vi "Check Reservation Groups Supported.vi"(8 "error in":errorcluster caption="error in (no error)") -> (0 "error out":errorcluster, 3 "use reservation groups?":bool)   [LabVIEW 2017, in "SLSC Switch Messaging.lvlib" / "SLSC Switch Consumer.lvclass"]
uses:
  SLSC Switch Consumer.lvclass
  <vilib>/nisyscfg/Get Installed Components.vi
  <vilib>/nisyscfg/Close (System).vi
  <vilib>/regexp/Match Regular Expression.xnode
  <vilib>/nisyscfg/nisyscfg.lvlib
  <vilib>/Utility/SystemLogging/NI_SystemLogging.lvlib
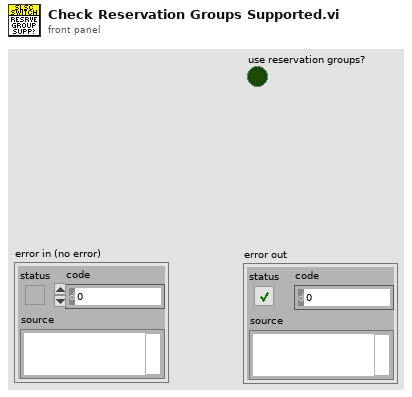
[diagram p1: front panel]
types:
  T1 = typedef "nisyscfg.lvlib/Software 1.2.ctl" = cluster{"title":string, "description":string, "ID":string, "version":string, "component type":T2}
  T2 = typedef "nisyscfg.lvlib/Component Type.ctl" = u32
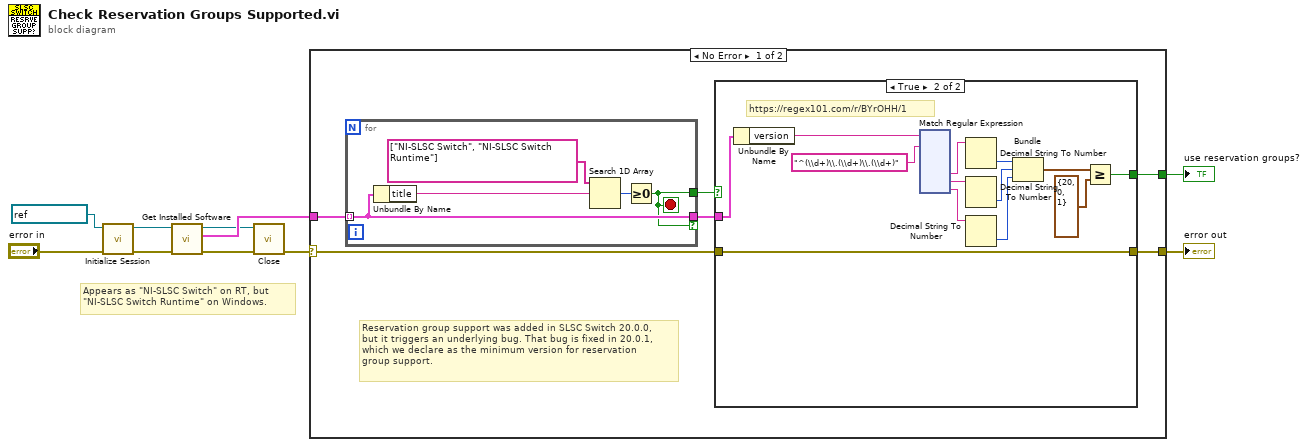
[diagram p0: block diagram]
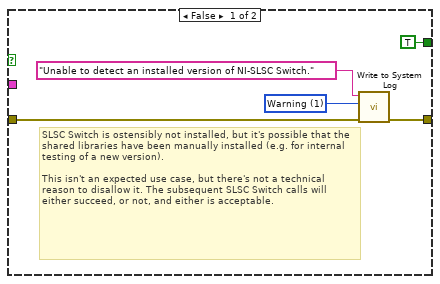
[diagram p2: hidden frame]
diagram:
  # "Appears as \"NI-SLSC Switch\" on RT, but\n\"NI-SLSC Switch Runtime\" on Windows."
  n1 = call <vilib>:"Initialize Session.vi"("error in (no error)"="error in", "Target (localhost)"=refnum<k21> "localhost") -> ("error out"=w9:errorcluster, "Session out"=w10:refnum<k21>)  [unwired: 8 in]
  n2 = call-poly <vilib>:"Get Installed Software.vi"("error in (no error)"=w9, "Session in"=w10) -> ("error out"=w6:errorcluster, "Software Components"=w8:T1[], "Session out"=w7:refnum<k21>)  [unwired: 7 in]
  n3 = call-poly <vilib>:"Close.vi"("error in (no error)"=w6, "Session in"=w7) -> ("error out"=w4:errorcluster)  [unwired: 9 in]
  n4 = case shown="No Error" w4 {
    selector: w4 -> [w12 w158]
    tunnel: w8 -> [w16 _]
    tunnel: [w13 _] -> w5
    tunnel: [w11 w158] -> w3
    frame No Error {
      # "Reservation group support was added in SLSC Switch 20.0.0,\nbut it triggers an underlying bug. That bug is fixed in 20.0.1,\nwhich we declare as the minimum version for reservation\ngroup support."
      n5 = for {
        tunnel: w16 -> [w157] mode=indexing
        tunnel: [w157] -> w14 if=w153
        tunnel: [w153] -> w15
        stop <- w153 stop-if-true
        n6 = Unbundle By Name(w157) -> ("title"=w155:string)
        n7 = Search 1D Array(1D array=string[] ["NI-SLSC Switch", "NI-SLSC Switch Runtime"], element=w155) -> (index of element=w154:i32)  [unwired: 1 in]
        n8 = Greater Or Equal To 0?(x=w154) -> (x >= 0?=w153:bool)
      }
      n9 = case shown="True" w15 {
        tunnel: [TRUE w26] -> w13
        tunnel: w14 -> [_ w27]
        tunnel: w12 -> [w19 w22]
        tunnel: [w18 w22] -> w11
        frame False {
          w20 = 1 items=["Error", "Warning", "Informational"] ("severity")
          # "SLSC Switch is ostensibly not installed, but it's possible that the shared libraries have been manually installed (e.g. for internal testing of a new version).\n\nThis isn't an expected use case, but there's not a technical reason to disallow it. The subsequent SLSC Switch calls will either succeed, or not, and either is acceptable."
          n10 = call <vilib>:"Write to System Log.vi"("error in (no error)"=w19, "severity"=w20, "message"="Unable to detect an installed version of NI-SLSC Switch.") -> ("error out"=w18:errorcluster)  [unwired: 8 in]
        }
        frame True {
          # "https://regex101.com/r/BYrOHH/1"
          n11 = Unbundle By Name(w27) -> ("version"=w23:string)
          n12 = xnode "Match Regular Expression"("input string"=w23, "regular expression"="^(\\d+)\\.(\\d+)\\.(\\d+)") -> ("submatch 1"=w29:string, "submatch 2"=w30:string, "submatch 3"=w31:string)  [unwired: 4 in, 5 out]
          n13 = Decimal String To Number(string=w29) -> (number=w32:i32)  [unwired: 2 in, 1 out]
          n14 = Decimal String To Number(string=w30) -> (number=w33:i32)  [unwired: 2 in, 1 out]
          n15 = Decimal String To Number(string=w31) -> (number=w34:i32)  [unwired: 2 in, 1 out]
          n16 = Bundle(w32, w33, w34) -> (w25:cluster{i32, i32, i32})  [unwired: 1 in]
          n17 = Greater Or Equal?(x=w25, y=cluster{i32, i32, i32} {20, 0, 1}) -> (x >= y?=w26:bool)
        }
      }
    }
    frame Error {
    }
  }
  "use reservation groups?" <- w5
  "error out" <- w3
